vi "Zernike Calculation.vi"(8 "error in (no error)":errorcluster, 10 "HasoSlopes in":refnum<class "HasoSlopes.lvclass">, 11 "HASO4_3 in":refnum<class "ILAO_BeamShaper.lvclass">) -> (0 "error out":errorcluster, 1 "Zernike Coefficients":sgl[](array[numeric]), 2 "HasoSlopes out":refnum<class "HasoSlopes.lvclass">, 3 "HASO4_3 out":refnum<class "ILAO_BeamShaper.lvclass">)   [LabVIEW 2020, in "ILAO_BeamShaper.lvclass"]
uses:
  ILAO_BeamShaper.lvclass
  HASO4_3/WaveKit/Classes/HasoSlopes/HasoSlopes.lvclass
  HASO4_3/WaveKit/Controls/Point2Df.ctl
  ILAO_BeamShaper.lvclass/ILAO_BeamShaper.ctl
  shared/CompressAndUpdate(Poly)/CompressAndUpdate(Numeric).vi
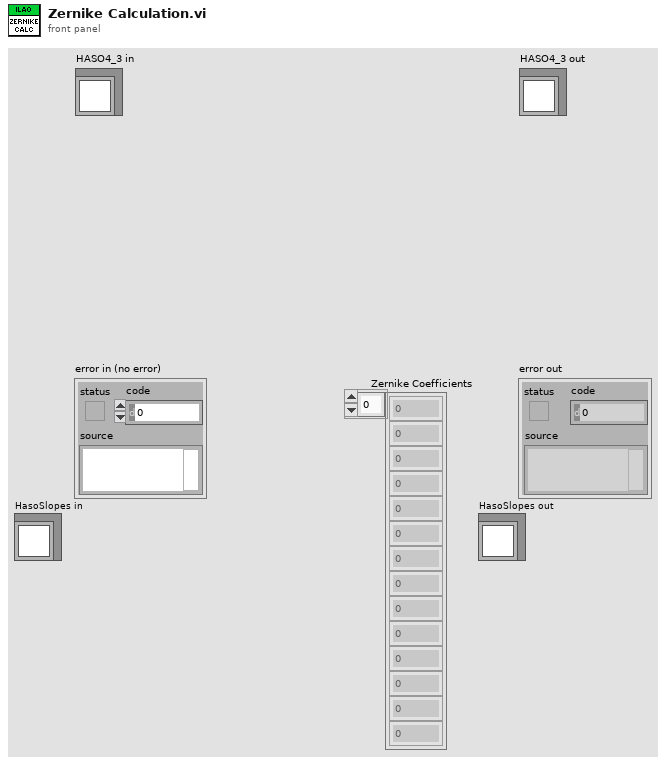
[diagram p1: front panel]
types:
  T1 = typedef "Point2Df.ctl" = cluster{"X":sgl, "Y":sgl}
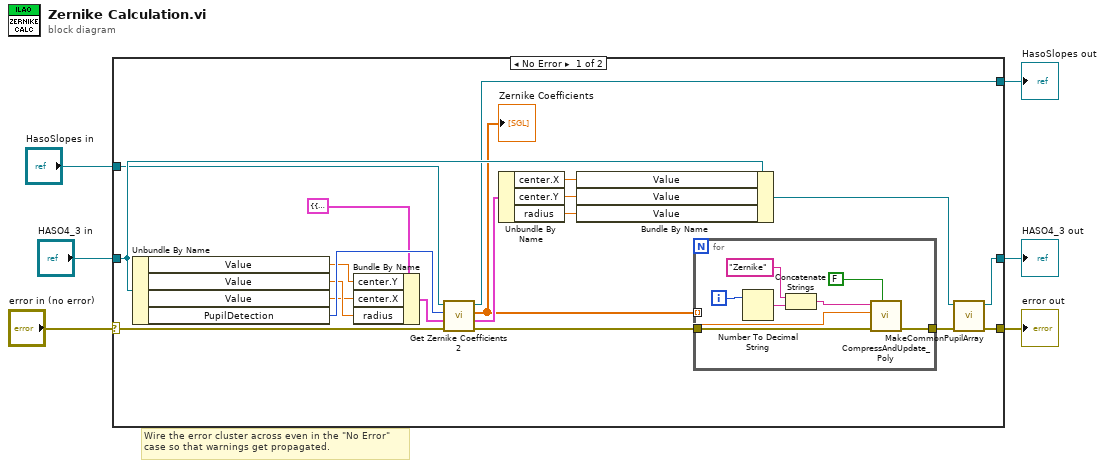
[diagram p0: block diagram]
diagram:
  # "Wire the error cluster across even in the \"No Error\"\ncase so that warnings get propagated."
  n1 = case shown="No Error" "error in (no error)" {
    selector: "error in (no error)" -> [w13 w37]
    tunnel: [w7 w37] -> w5
    tunnel: [w8 w36] -> w3
    tunnel: "HASO4_3 in" -> [w20 w36]
    tunnel: "HasoSlopes in" -> [w15 w35]
    tunnel: [w14 w35] -> w1
    frame No Error {
      n2 = Unbundle By Name(w20) -> ("Value"=w23:dbl, "Value"=w25:dbl, "Value"=w24:dbl, "PupilDetection"=w26:enum16{"Manual", "Automatic"})
      n3 = Bundle By Name(cluster=cluster{"center":T1, "radius":sgl} {"center"={"X"=0.0, "Y"=0.0}, "radius"=0.0} ("Pupil"), "center.Y"=w23, "center.X"=w24, "radius"=w25) -> (w22:cluster{"center":T1, "radius":sgl})
      n4 = call "Get Zernike Coefficients 2.vi"("error in (no error)"=w13, "Pupil"=w22, "PupilDetectionOption"=w26, "HasoSlopes in"=w15) -> ("error out"=w11:errorcluster, "Pupil out"=w19:cluster{"center":T1, "radius":sgl}, "Zernike Coefficients"=w12:dbl[], "HasoSlopes out"=w14:refnum<class "HasoSlopes.lvclass">)  [unwired: 4 in]
      "Zernike Coefficients" <- w12
      n5 = Unbundle By Name(w19) -> ("center.X"=w18:sgl, "center.Y"=w17:sgl, "radius"=w16:sgl)
      n6 = Bundle By Name(cluster=w20, "Value"=w18, "Value"=w17, "Value"=w16) -> (w10:refnum<class "ILAO_BeamShaper.lvclass">)
      n7 = for {
        tunnel: w12 -> [w34] mode=indexing
        tunnel: w11 -> [w28]
        tunnel: [w27] -> w9
        i -> [w32]
        n8 = Number To Decimal String(number=w32) -> (decimal integer string=w31:string)  [unwired: 1 in]
        n9 = Concatenate Strings("Zernike" ("command or variable name"), w31) -> (w30:string)
        n10 = call-poly "CompressAndUpdate_Poly.vi"("force CVT update (false)"=FALSE, "error in"=w28, "Numeric"=w34, "command or variable name"=w30) -> ("error out"=w27:errorcluster)  [unwired: 7 in]
      }
      n11 = call-dynamic "MakeCommonPupilArray.vi"("error in (no error)"=w9, "HASO4_3 in"=w10) -> ("error out"=w7:errorcluster, "HASO4_3 out"=w8:refnum<class "ILAO_BeamShaper.lvclass">)  [unwired: 8 in]
    }
    frame Error {
    }
  }
  "error out" <- w5
  "HASO4_3 out" <- w3
  "HasoSlopes out" <- w1
